vi "WavPlay.vi"(8 "error in (no error)":errorcluster, 10 "OkNg":enum16{"OK", "NG", "NG1", "SCAN"}(ring), 11 "Device ID":u32) -> (0 "error out":errorcluster)   [LabVIEW 2014]
panel:
  in  "path":path=path "C:/AC-BarCode/sound/test.wav"
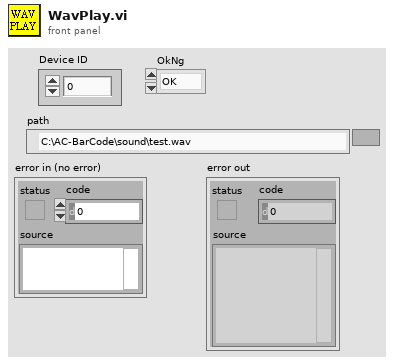
[diagram p1: front panel]
types:
  T1 = typedef "Sound Output Task ID.ctl" = u32
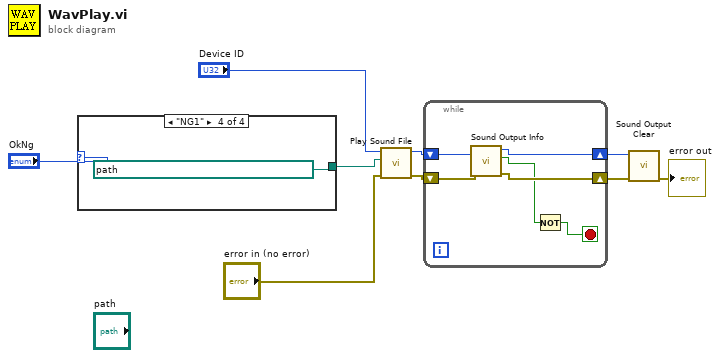
[diagram p0: block diagram]
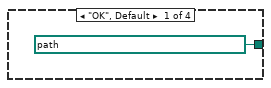
[diagram p2: hidden frame]
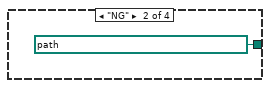
[diagram p3: hidden frame]
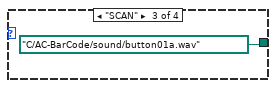
[diagram p4: hidden frame]
diagram:
  n1 = case shown="\"NG1\"" "OkNg" {
    tunnel: [path "C:/AC-BarCode/sound/照合OK.wav" ("path") path "C:/AC-BarCode/sound/照合NG.wav" ("path") path "C:/AC-BarCode/sound/button01a.wav" ("path") path "C:/AC-BarCode/sound/照合NG2.wav" ("path")] -> w1
    frame "OK", Default {
    }
    frame "NG" {
    }
    frame "SCAN" {
    }
    frame "NG1" {
    }
  }
  n2 = call <vilib>:"Play Sound File.vi"("error in (no error)"="error in (no error)", "path"=w1, "device ID"="Device ID") -> ("error out"=w8:errorcluster, "task ID"=w9:T1)  [unwired: 7 in]
  n3 = while {
    shift-right: [w17] -> w7
    shift-left: w9 -> [w19]
    shift-right: [w16] -> w6
    shift-left: w8 -> [w18]
    stop <- w14 stop-if-true
    n4 = call <vilib>:"Sound Output Info.vi"("error in (no error)"=w18, "task ID"=w19) -> ("error out"=w16:errorcluster, "is playing?"=w15:bool, "task ID out"=w17:T1)  [unwired: 6 in, 1 out]
    n5 = Not(x=w15) -> (.not. x?=w14:bool)
  }
  n6 = call <vilib>:"Sound Output Clear.vi"("error in (no error)"=w6, "task ID"=w7) -> ("error out"=→"error out":errorcluster)  [unwired: 9 in]
